vi "DraggingDresser.vi"() -> ()   [LabVIEW 2014]
panel:
  in  "Coefficient of Kinetic Friction":dbl min=0.0 max=1.0
  out "Force":dbl[](array[numeric])
  out "Angle for Minimum Force":i32 format="%.1f"
  out "Waveform Graph":dbl[](graph)
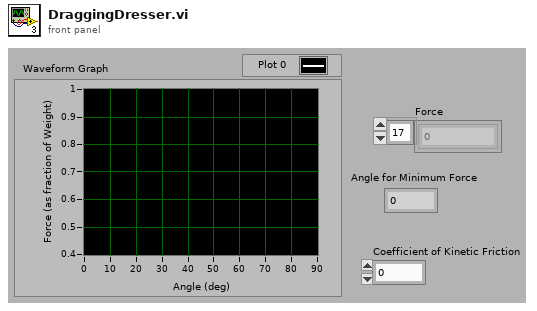
[diagram p1: front panel]
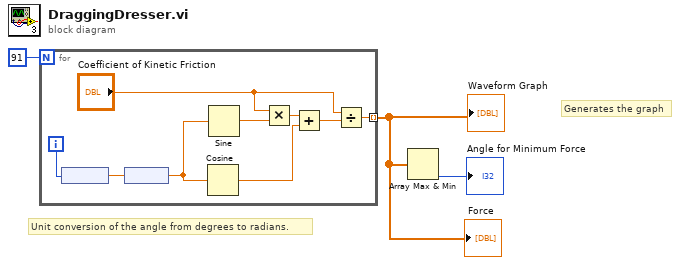
[diagram p0: block diagram]
diagram:
  # "Generates the graph"
  # "Unit conversion of the angle from degrees to radians."
  n1 = for {
    N: 91 -> [_]
    tunnel: [w8] -> w1 mode=indexing
    i -> [w6]
    n2 = node(w6) -> (w7:dbl[unit])
    n3 = node(w7) -> (w5:dbl)
    n4 = Cosine(x=w5) -> (cos(x)=w10:dbl)
    n5 = Sine(x=w5) -> (sin(x)=w12:dbl)
    n6 = Multiply(x="Coefficient of Kinetic Friction", y=w12) -> (x*y=w11:dbl)
    n7 = Add(x=w11, y=w10) -> (x+y=w9:dbl)
    n8 = Divide(x="Coefficient of Kinetic Friction", y=w9) -> (x/y=w8:dbl)
  }
  "Waveform Graph" <- w1
  "Force" <- w1
  n9 = Array Max & Min(array=w1) -> (min index (indices)=→"Angle for Minimum Force":i32)  [unwired: 3 out]
